vi "DRAM Bank0 Read Write (SubVI).vi"   [LabVIEW 2015]
uses:
  Image Compression/SubVIs (FPGA)/DRAM Read.ctl
  <vilib>/rvi/eio/common/nirviEmuTemplateMethod_errors.vi
  <vilib>/rvi/Emulation/niFpgaEmulationIsFPGAContextNoSignature.vi
  <vilib>/rvi/Emulation/niFpgaSctlEmulationGetInTimedLoop.vi
  <vilib>/rvi/errors/niFpgaSetErrorForExecOnDevCompSimple.vi
  <vilib>/rvi/eio/common/nirviEmuReportErrorAndStop.vi
  <vilib>/rvi/DataTransferAndStorage/Container/Common/niFpgaContainerGetUniqueNameForEmu.vi
  <vilib>/rvi/FIFO/Fifo_Resource/nirvififoEmulationSetSize.vi
  <vilib>/rvi/FIFO/Fifo_Resource/nirviFifoEmulationQueueMgr.vi
  <instcachedir>/0/nirviFifoEmulationQueueMgr_E5CAEC123FF24DC58D834DCA3CDAA9B5.lvgen/nirviFifoEmulationQueueMgr_E5CAEC123FF24DC58D834DCA3CDAA9B5_006.vi
  <vilib>/Utility/error.llb/Clear Errors.vi
  <vilib>/rvi/FIFO/Fifo_Resource/nirvififoEmulationCreateLock.vi
  <vilib>/rvi/Emulation/niFpgaProcessEmulError.vi
  <vilib>/rvi/FIFO/Fifo_Resource/nirvififoEmulationObtainLock.vi
  <vilib>/rvi/FIFO/Fifo_Resource/nirvififoEmulationReleaseLock.vi
  <vilib>/rvi/occurrence/nirviWaitOnOccurrenceBase.vi
  <vilib>/rvi/errors/nirviReportUnexpectedCaseInternalError.vi
  <vilib>/rvi/errors/nirviReportUnexpectedCaseInternalError (U32).vi
  <vilib>/rvi/FIFO/Fifo_Resource/nirvififoEmulationDetermineInputValidOut.vi
  <vilib>/eio/EIONode/EIONode.xnode
  <vilib>/rvi/DataTransferAndStorage/Container/XNode/niFpgaContainer.xnode
  <vilib>/rvi/FIFO/Fifo_Resource/nirvififoEmulationRead.vi
  <vilib>/rvi/FIFO/Fifo_Resource/nirvififoEmulationGetNumberOfElementsToWrite.vi
  <vilib>/rvi/FIFO/Fifo_Resource/nirvififoEmulationWrite.vi
types:
  T1 = typedef "DRAM Read.ctl" = enum16{"Clear FIFO", "Read"}
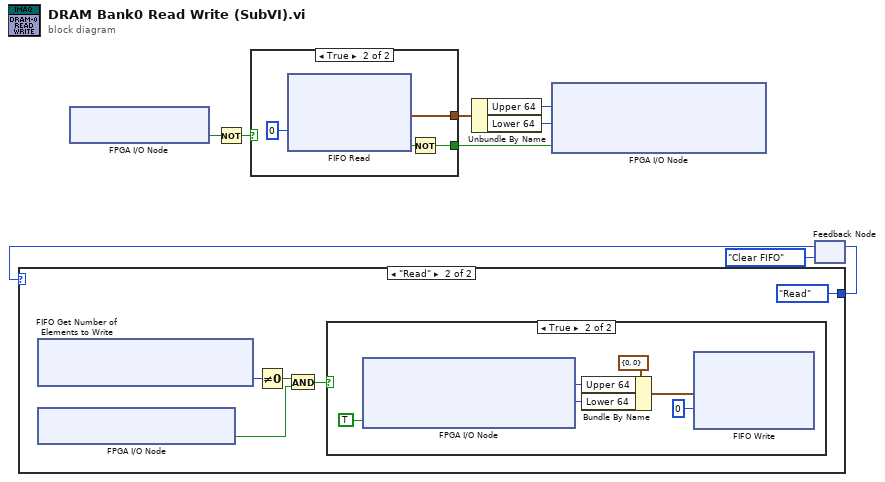
[diagram p0: block diagram]
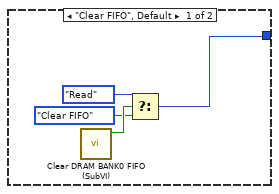
[diagram p2: hidden frame]
diagram:
  n1 = xnode "FPGA I/O Node"() -> ("DRAM Bank 0\\Full"=w4:bool)  [unwired: 1 in, 1 out]
  n2 = Not(x=w4) -> (.not. x?=w5:bool)
  n3 = case shown="True" w5 {
    tunnel: [_ w12] -> w7
    tunnel: [_ w10] -> w6
    frame False {
    }
    frame True {
      n4 = xnode ("FIFO Read")("Timeout"=0) -> ("Element"=w12:cluster{"Lower 64":u64, "Upper 64":u64}, "Timed Out?"=w11:bool)  [unwired: 1 in, 1 out]
      n5 = Not(x=w11) -> (.not. x?=w10:bool)
    }
  }
  n6 = Unbundle By Name(w7) -> ("Upper 64"=w8:u64, "Lower 64"=w9:u64)
  n7 = xnode "FPGA I/O Node"("DRAM Bank 0\\Write_Data_Upper"=w8, "DRAM Bank 0\\Write_Data_Lower"=w9, "DRAM Bank 0\\Write"=w6) -> ()  [unwired: 3 in, 3 out]
  n8 = feedback #1(DRAM_Read."Clear FIFO" ("f")) -> (w2:T1)
  n9 = case shown="\"Clear FIFO\", Default" w2 {
    tunnel: [w15 DRAM_Read."Read" ("f")] -> w3
    frame "Clear FIFO", Default {
      n10 = call "Clear DRAM BANK0 FIFO (SubVI).vi"() -> ("DRAM FIFO Clear?"=w17:bool)  [unwired: 11 in]
      n11 = Select(t=DRAM_Read."Read", s=w17, f=DRAM_Read."Clear FIFO") -> (s? t:f=w15:T1)
    }
    frame "Read" {
      n12 = xnode ("FIFO Get Number of Elements to Write")() -> ("Number of Elements to Write"=w19:u32)  [unwired: 1 in, 1 out]
      n13 = xnode "FPGA I/O Node"() -> ("DRAM Bank 0\\Data_Available"=w21:bool)  [unwired: 1 in, 1 out]
      n14 = Not Equal To 0?(x=w19) -> (x != 0?=w20:bool)
      n15 = And(x=w20, y=w21) -> (x .and. y?=w22:bool)
      n16 = case shown="True" w22 {
        frame False {
        }
        frame True {
          n17 = xnode "FPGA I/O Node"("DRAM Bank 0\\Read"=TRUE ("DRAM Bank 0\\Read")) -> ("DRAM Bank 0\\Read_Data_Upper"=w25:u64, "DRAM Bank 0\\Read_Data_Lower"=w24:u64)  [unwired: 3 in, 3 out]
          n18 = Bundle By Name(cluster=cluster{"Lower 64":u64, "Upper 64":u64} {"Lower 64"=0, "Upper 64"=0} ("Element"), "Upper 64"=w25, "Lower 64"=w24) -> (w23:cluster{"Lower 64":u64, "Upper 64":u64})
          n19 = xnode ("FIFO Write")("Element"=w23, "Timeout"=0) -> ()  [unwired: 1 in, 2 out]
        }
      }
    }
  }
  n20 = feedback-in #1(w3) -> ()
